vi "F Dwf Get Version.vi"(8 "error in (no error)":errorcluster, 11 "szVersion":string) -> (0 "error out":errorcluster, 2 "function return":i32, 3 "szVersion out":string)   [LabVIEW 2019, in "Olasdwf.lvlib"]
doc: "DWFAPI int FDwfGetVersion(char szVersion[32]);"
uses:
  Olasdwf.lvlib
  Windows/System32/dwf.dll
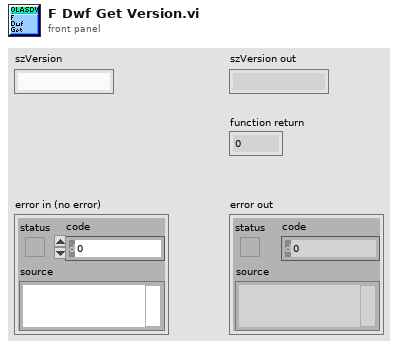
[diagram p1: front panel]
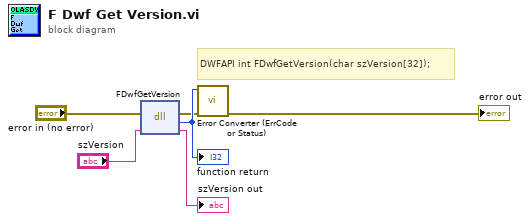
[diagram p0: block diagram]
diagram:
  # "DWFAPI int FDwfGetVersion(char szVersion[32]);"
  n1 = dll-call lib="C:/Windows/System32/dwf.*" fn="FDwfGetVersion"(error in="error in (no error)", "szVersion"="szVersion") -> (error out=w2:errorcluster, w6:i32, "szVersion"=→"szVersion out":string)  [unwired: 2 in, 1 out]
  "function return" <- w6
  n2 = call "Error Converter (ErrCode or Status).vi"("error in (no error)"=w2, "error code"=w6) -> ("error out"=→"error out":errorcluster)  [unwired: 9 in]
